vi "Destroy.vi"(0 "reference":refnum<class "ChoiceNode.lvclass">, 5 "error in (no error)":errorcluster) -> (15 "# of objects":i32, 19 "error out":errorcluster)   [LabVIEW 2014, in "ChoiceNode.lvclass"]
doc: "Destroys a StateNode object created with a StateNode constructor VI.\n\n[GOOP 2.1]"
uses:
  <resource>/Framework/Providers/Open_GDS/UML/ChoiceNode_class/ChoiceNode.lvclass
  <resource>/Framework/Providers/Open_GDS/UML/RectangularNode_class/RectangularNode.lvclass
  <resource>/Framework/Providers/Open_GDS/UML/MultiLineString_class/MultiLineString.lvclass
panel:
  out "reference out":refnum<class "ChoiceNode.lvclass">
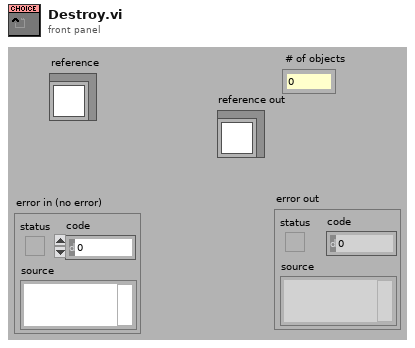
[diagram p1: front panel]
types:
  T1 = typedef "ChoiceNode.lvclass/ObjectAttributes.ctl" = cluster{"Text":refnum<class "MultiLineString.lvclass">, "DEFAULT_WIDTH":i32, "DEFAULT_HEIGHT":i32}
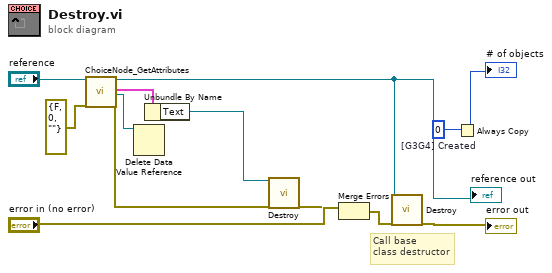
[diagram p0: block diagram]
diagram:
  w1 = 0  # [G3G4] Created
  # "Call base\nclass destructor"
  n1 = call <resource>:"ChoiceNode_GetAttributes.vi"("reference in"="reference", "error in (no error)"=errorcluster {"status"=FALSE, "code"=0, "source"=""}) -> ("reference out"=w7:refnum<class "ChoiceNode.lvclass">, "Data"=w4:T1, "DataRef"=w3:refnum<data-value>, "error out"=w5:errorcluster)  [unwired: 1 in, 13 out]
  "reference out" <- w7
  n2 = Delete Data Value Reference(data value reference=w3) -> ()  [unwired: 1 in, 2 out]
  n3 = Unbundle By Name(w4) -> ("Text"=w9:refnum<class "MultiLineString.lvclass">)
  n4 = call-dynamic "Destroy.vi"("reference"=w9, "error in (no error)"=w5) -> ("error out"=w8:errorcluster)  [unwired: 16 in, 1 out]
  n5 = Merge Errors("error in (no error)", w8) -> (w6:errorcluster)
  n6 = call-parent "Destroy.vi"("reference"=w7, "error in (no error)"=w6) -> ("error out"=→"error out":errorcluster)  [unwired: 16 in, 1 out]
  n7 = Always Copy(1:w1) -> (0:→"# of objects":i32)
